vi "DSW Density of Saline Water(Kg to m^3).vi"(1 "Salinity":dbl, 2 "Sailne Water Temprature":dbl[unit]) -> (0 "DSW":dbl[unit])   [LabVIEW 2018]
panel:
  out "Saline Water Temprature":dbl[unit](slide) scale=0.0..100.0
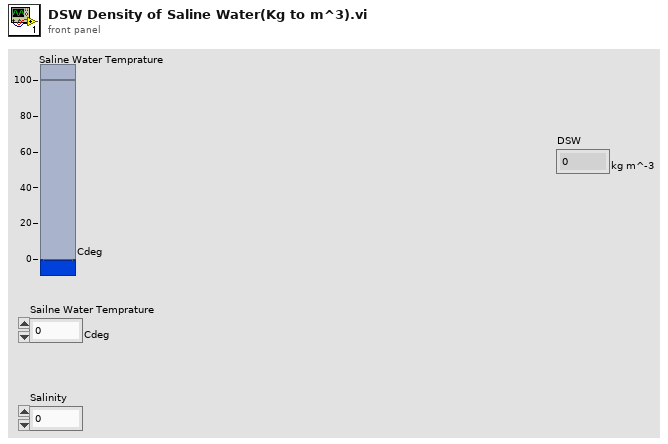
[diagram p1: front panel]
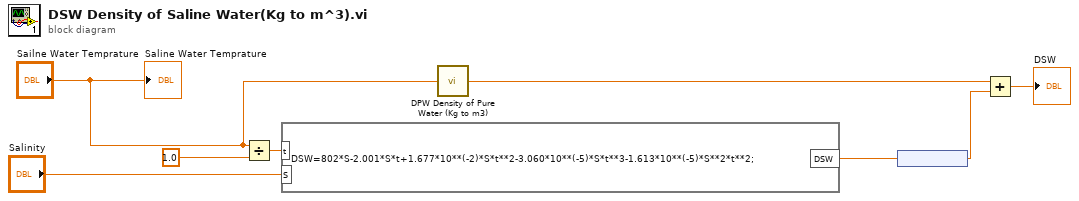
[diagram p0: block diagram]
diagram:
  n1 = Divide(x="Sailne Water Temprature", y=dbl[unit] 1.0) -> (x/y=w8:dbl)
  n2 = formula code="DSW=802*S-2.001*S*t+1.677*10**(-2)*S*t**2-3.060*10**(-5)*S*t**3-1.613*10**(-5)*S**2*t**2;"("t"=w8, "S"="Salinity") -> ("DSW"=w1:dbl)
  n3 = call "DPW Density of Pure Water (Kg to m3).vi"("Pure Water Temprature"="Sailne Water Temprature") -> ("DPW"=w3:dbl[unit])
  n4 = node(w1) -> (w4:dbl[unit])
  n5 = Add(x=w3, y=w4) -> (x+y=→"DSW":dbl[unit])
  "Saline Water Temprature" <- "Sailne Water Temprature"
